vi "Save Debug Snapshot.vi"(6 "IPath Getter in":refnum<class "IPath Getter.lvclass">, 7 "Debug Elements Options":T1={"Breakpoints"=TRUE, "Probes"=TRUE}, 8 "error in":errorcluster, 9 "Probes":i32[](array[numeric]), 10 "Breakpoints":T2[](array[typedef]), 11 "VI Reference in":refnum<vi>) -> (0 "error out":errorcluster, 3 "VI Reference out":refnum<vi>)   [LabVIEW 2020]
doc: "Save <b>Debug Snapshot</b> of the active VI to the Cache File."
uses:
  Type Definitions/Breakpoint--cluster.ctl
  <vilib>/Utility/miscctls.llb/LVBreakpointStatusEnum.ctl
  Type Definitions/Class Name--enum.ctl
  Type Definitions/Snapshot Handling Options--cluster.ctl
  IPath Getter/IPath Getter.lvclass
  Type Definitions/Debug Snapshot--cluster.ctl
  Type Definitions/Debug Snapshot Array--cluster.ctl
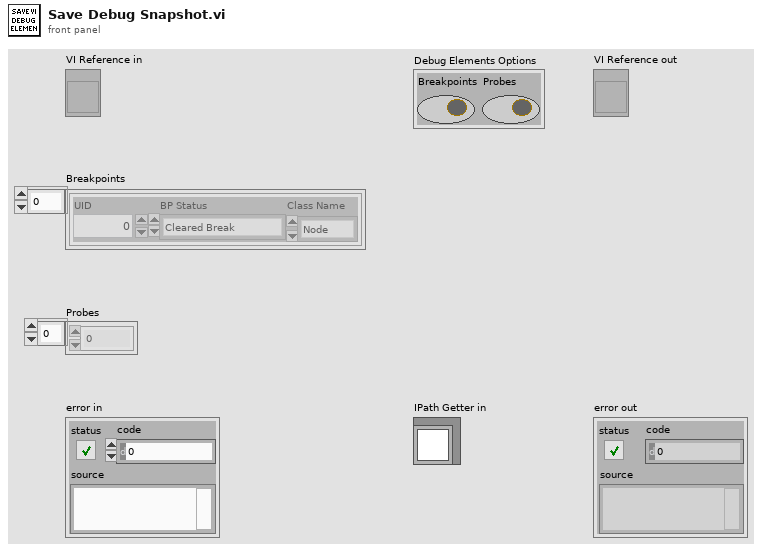
[diagram p1: front panel]
types:
  T1 = typedef "Snapshot Handling Options--cluster.ctl" = cluster{"Breakpoints":bool, "Probes":bool}
  T2 = typedef "Breakpoint--cluster.ctl" = cluster{"UID":i32, "BP Status":T3, "Class Name":T4}
  T3 = typedef "LVBreakpointStatusEnum.ctl" = enum8{"Cleared Break", "Enabled Break", "Disabled Break"}
  T4 = typedef "Class Name--enum.ctl" = enum16{"Node", "Wire"}
  T5 = typedef "Debug Snapshot Array--cluster.ctl" = cluster{"Debug Snapshots":T6[]}
  T6 = typedef "Debug Snapshot--cluster.ctl" = cluster{"VI Name":string, "Breakpoints":T2[], "Probes":i32[]}
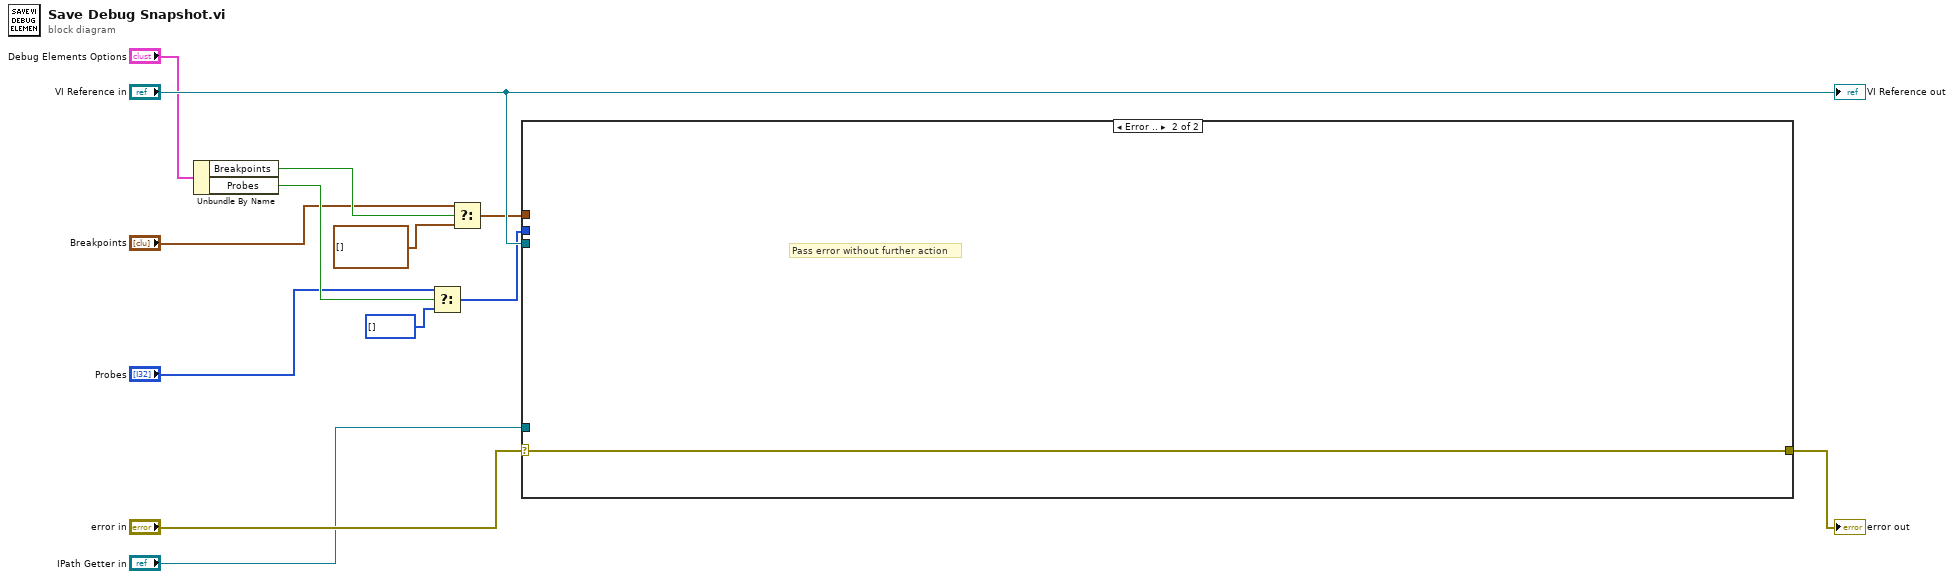
[diagram p0: block diagram]
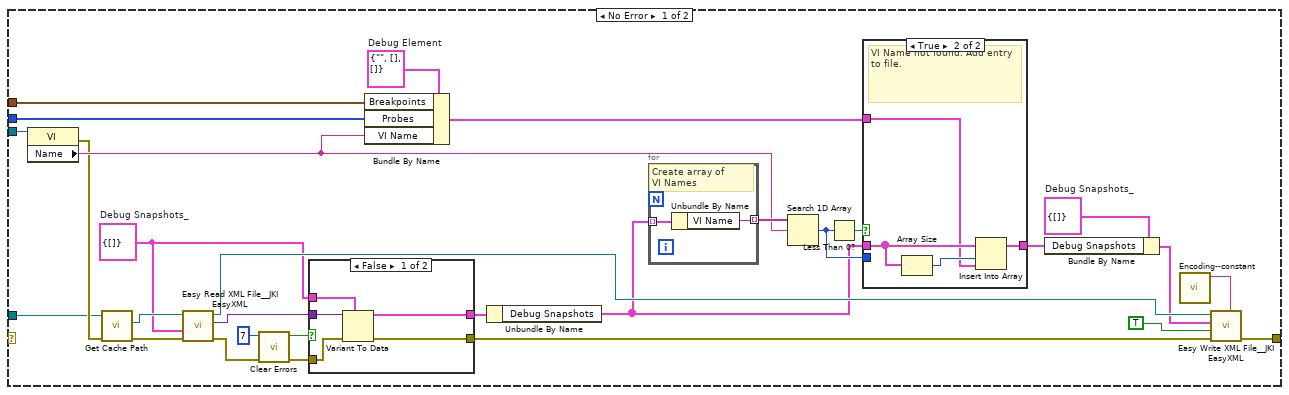
[diagram p2: hidden frame]
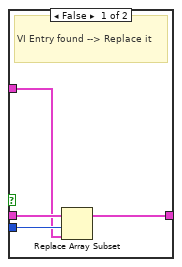
[diagram p4: hidden frame]
diagram:
  n1 = Unbundle By Name("Debug Elements Options") -> ("Breakpoints"=w9:bool, "Probes"=w8:bool)
  n2 = Select(t="Probes", s=w8, f=i32[] []) -> (s? t:f=w2:i32[])
  n3 = Select(t="Breakpoints", s=w9, f=T2[] []) -> (s? t:f=w3:T2[])
  n4 = case shown="Error .." "error in" {
    selector: "error in" -> [_ w59]
    tunnel: w3 -> [w40 _]
    tunnel: [w38 w59] -> w12
    tunnel: "VI Reference in" -> [w42 _]
    tunnel: w2 -> [w37 _]
    tunnel: "IPath Getter in" -> [w20 _]
    frame No Error {
      w16 = T5 {"Debug Snapshots"=[]}  # Debug Snapshots_
      w19 = T5 {"Debug Snapshots"=[]}  # Debug Snapshots_
      w41 = T6 {"VI Name"="", "Breakpoints"=[], "Probes"=[]}  # Debug Element
      n5 = property class="VI"(reference=w42) -> (error out=w23:errorcluster, "Name"=w31:string)  [unwired: 1 in, 1 out]
      n6 = call-dynamic "Get Cache Path.vi"("error in (no error)"=w23, "IPath Getter in"=w20) -> ("error out"=w22:errorcluster, "Path"=w21:path)  [unwired: 8 in]
      n7 = call <vilib>:"Easy Read XML File__JKI EasyXML.vi"("error in (no error)"=w22, "LabVIEW Data (Type)"=w19, "XML File Path"=w21) -> ("error out"=w26:errorcluster, "LabVIEW Data"=w36:variant, "XML File Path (duplicate)"=w29:path)  [unwired: 6 in]
      n8 = call <vilib>:"Clear Errors.vi"("error in (no error)"=w26, "specific error code to clear (0: all)"=7) -> ("error out"=w25:errorcluster, "specific error cleared?"=w24:bool)  [unwired: 4 in]
      n9 = case shown="False" w24 {
        tunnel: w36 -> [w47 _]
        tunnel: w19 -> [w46 _]
        tunnel: [w45 _] -> w18
        tunnel: [w44 w48] -> w30
        tunnel: w25 -> [w43 w48]
        frame False {
          n10 = Variant To Data(error in=w43, type=w46, Variant=w47) -> (data=w45:T5, error out=w44:errorcluster)
        }
        frame True {
        }
      }
      n11 = Bundle By Name(cluster=w41, "Breakpoints"=w40, "Probes"=w37, "VI Name"=w31) -> (w33:T6)
      n12 = Unbundle By Name(w18) -> ("Debug Snapshots"=w17:T6[])
      n13 = for {
        tunnel: [w58] -> w35 mode=indexing
        tunnel: w17 -> [w57] mode=indexing
        # "Create array of\nVI Names"
        n14 = Unbundle By Name(w57) -> ("VI Name"=w58:string)
      }
      n15 = Search 1D Array(1D array=w35, element=w31) -> (index of element=w32:i32)  [unwired: 1 in]
      n16 = Less Than 0?(x=w32) -> (x < 0?=w34:bool)
      n17 = case shown="True" w34 {
        tunnel: w17 -> [w52 w56]
        tunnel: w33 -> [w50 w54]
        tunnel: [w49 w53] -> w15
        tunnel: w32 -> [w51 _]
        frame False {
          # "VI Entry found --> Replace it"
          n18 = Replace Array Subset(array=w52, new element=w50, index=w51) -> (w49:T6[])
        }
        frame True {
          # "VI Name not found. Add entry to file."
          n19 = Array Size(array=w56) -> (size(s)=w55:i32)
          n20 = Insert Into Array(array=w56, index=w55, new element=w54) -> (w53:T6[])
        }
      }
      n21 = Bundle By Name(cluster=w16, "Debug Snapshots"=w15) -> (w14:T5)
      n22 = call "Encoding--constant.vi"() -> ("Encoding (none)"=w39:string)  [unwired: 11 in]
      n23 = call <vilib>:"Easy Write XML File__JKI EasyXML.vi"("Encoding (none)"=w39, "error in (no error)"=w30, "Overwrite File? (false)"=TRUE, "LabVIEW Data"=w14, "XML File Path"=w29) -> ("error out"=w38:errorcluster)  [unwired: 5 in, 1 out]
    }
    frame Error {
      # "Pass error without further action"
    }
  }
  "error out" <- w12
  "VI Reference out" <- "VI Reference in"
